vi "Main HMI.vi"() -> ()   [LabVIEW 2014]
uses:
  Controls/Icon Arrow H.ctl
  Controls/Icon Line H.ctl
  Controls/Icon Switch H.ctl
  Controls/Meter SOC.ctl
  Controls/Icon Load.ctl
  Controls/Icon Battery.ctl
  Controls/Icon Inverter.ctl
  Controls/Icon Generator.ctl
  Controls/Icon PV.ctl
  Controls/HMI Tab.ctl
  Controls/Alarm Display.ctl
  Controls/Icon Line V.ctl
  Controls/Icon Arrow V.ctl
  Controls/Icon Switch V.ctl
  Controls/Interface Data.ctl
  Controls/Gen Data.ctl
  Controls/HMI State.ctl
  Controls/Alarms Data.ctl
  Controls/LogState.ctl
panel:
  out "Alarms Page":bool=TRUE
  out "Main Page":bool=TRUE
  out "Tab Control":T1
  out "Arrow 2":T2
  out "Arrow 1":T2
  out "Line Inverter3":T3
  out "Line Inverter2":T4
  out "Arrow 19":T5
  out "Arrow 18":T5
  out "Arrow 17":T5
  out "Arrow 16":T5
  out "Arrow 15":T5
  out "Arrow 12":T5
  out "Arrow 11":T5
  out "Line Gen Both":T4
  out "Line Inverter1":T3
  out "Line Gen W 3":T4
  out "Line Gen E 4":T4
  out "SOH":dbl format="%2.0f %"
  out "Gen East Hours":dbl format="%2.0f Hrs"
  out "Switch Gen E":T6
  out "Gen West Hours":dbl format="%2.0f Hrs"
  out "Gen East":T7
  out "Line Gen E 2":T4
  out "Load":T8
  out "Line Load":T4
  out "Arrow 10":T5
  out "Arrow 9":T5
  out "Switch Gen W":T6
  out "Switch Battery":T6
  out "Line Gen W 2":T4
  out "Gen West":T7
  out "SOC":T9 scale=0.0..100.0 scale format="%3.0f %"
  out "Batteries":T10
  out "Inverter":T11
  out "Line Batteries 1":T4
  out "Line Batteries 2":T4
  out "Switch PV":T6
  out "PV":T12
  out "Line PV":T4
  out "Line PV2":T4
  out "Solar kW":dbl format="%2.1f kW"
  out "Line Gen E 3":T3
  out "Line PV3":T3
  out "Switch Inverter":T13
  out "Converter Version":string
  out "RT Version":string
  out "FPGA Version":string
  out "HMI Version":string
  in  "Exit Program":bool
  out "InterfaceData":T14 {"GenEast"."TotalFuel(L)" format="%.2f"; "GenEast"."FuelRate(L/H)" format="%.2f"; "GenEast"."ApparentPower(VA)" format="%.2f"; "GenEast"."BattVoltage(V)" format="%.2f"; "GenEast"."Freq(Hz)" format="%.2f"; "GenEast"."RunHours(hr)" format="%.2f"; "GenEast"."PowerFactor" format="%.2f"; "GenEast"."ReactivePower(VAR)" format="%.2f"; "GenEast"."ActivePower(W)" format="%.2f"; "GenWest"."TotalFuel(L)" format="%.2f"; "GenWest"."FuelRate(L/H)" format="%.2f"; "GenWest"."ApparentPower(VA)" format="%.2f"; "GenWest"."BattVoltage(V)" format="%.2f"; "GenWest"."Freq(Hz)" format="%.2f"; "GenWest"."RunHours(hr)" format="%.2f"; "GenWest"."PowerFactor" format="%.2f"; "GenWest"."ReactivePower(VAR)" format="%.2f"; "GenWest"."ActivePower(W)" format="%.2f"; "Converter Alarms 2" format="%016b"; "Converter Faults 2" format="%016b"; "Controller Faults" format="%016b"; "System Status" format="%016b"; "Converter Alarms 1" format="%016b"; "Converter Faults 1" format="%016b"; "Solar Faults" format="%016b"; "ES Rack 10 Alarms" format="%016b"; "ES Rack 9 Alarms" format="%016b"; "ES Rack 8 Alarms" format="%016b"; "ES Rack 7 Alarms" format="%016b"; "ES Rack 6 Alarms" format="%016b"; "ES Rack 5 Alarms" format="%016b"; "ES Rack 4 Alarms" format="%016b"; "ES Rack 3 Alarms" format="%016b"; "ES Rack 2 Alarms" format="%016b"; "ES Rack 1 Alarms" format="%016b"; "ES System Alarms" format="%016b"; "System Faults" format="%016b"; "ES Rack 10 Faults" format="%016b"; "ES Rack 9 Faults" format="%016b"; "ES Rack 8 Faults" format="%016b"; "ES Rack 7  Faults" format="%016b"; "ES Rack 6 Faults" format="%016b"; "ES Rack 5 Faults" format="%016b"; "ES Rack 4 Faults" format="%016b"; "ES Rack 3 Faults" format="%016b"; "ES Rack 2 Faults" format="%016b"; "ES Rack 1 Faults" format="%016b"; "ES System Faults" format="%016b"}
  out "Alarms List":T16
  in  "Clear Alarms":bool
  out "Event Log Error":bool
  out "Data Log Error":bool
  out "GENERATOR EAST":T17(ring)
  out "GENERATOR WEST":T17(ring)
  out "POWER SYSTEM STATUS":T18(ring)
  out "SOLAR ARRAY":T19(ring)
  out "BATTERY ARRAY":T17(ring)
  out "Status Page":bool=TRUE
  out "Connection Error":bool
  out "System Status":string
  out "Diagnostics Page":bool=TRUE
  out "Fault Banner":bool
  out "Alarm Banner":bool
  # "Manual\nBreaker"
  # "Manual\nBreaker"
  # "Manual\nBreaker"
  # "Facility"
  # "Manual\nBreaker"
  # "Service Entrance Switchboard"
  # "Generator Housing"
  # "Solar Array Box"
  # "Manual\nBreaker"
  # "Battery Connex/Solid State Generator"
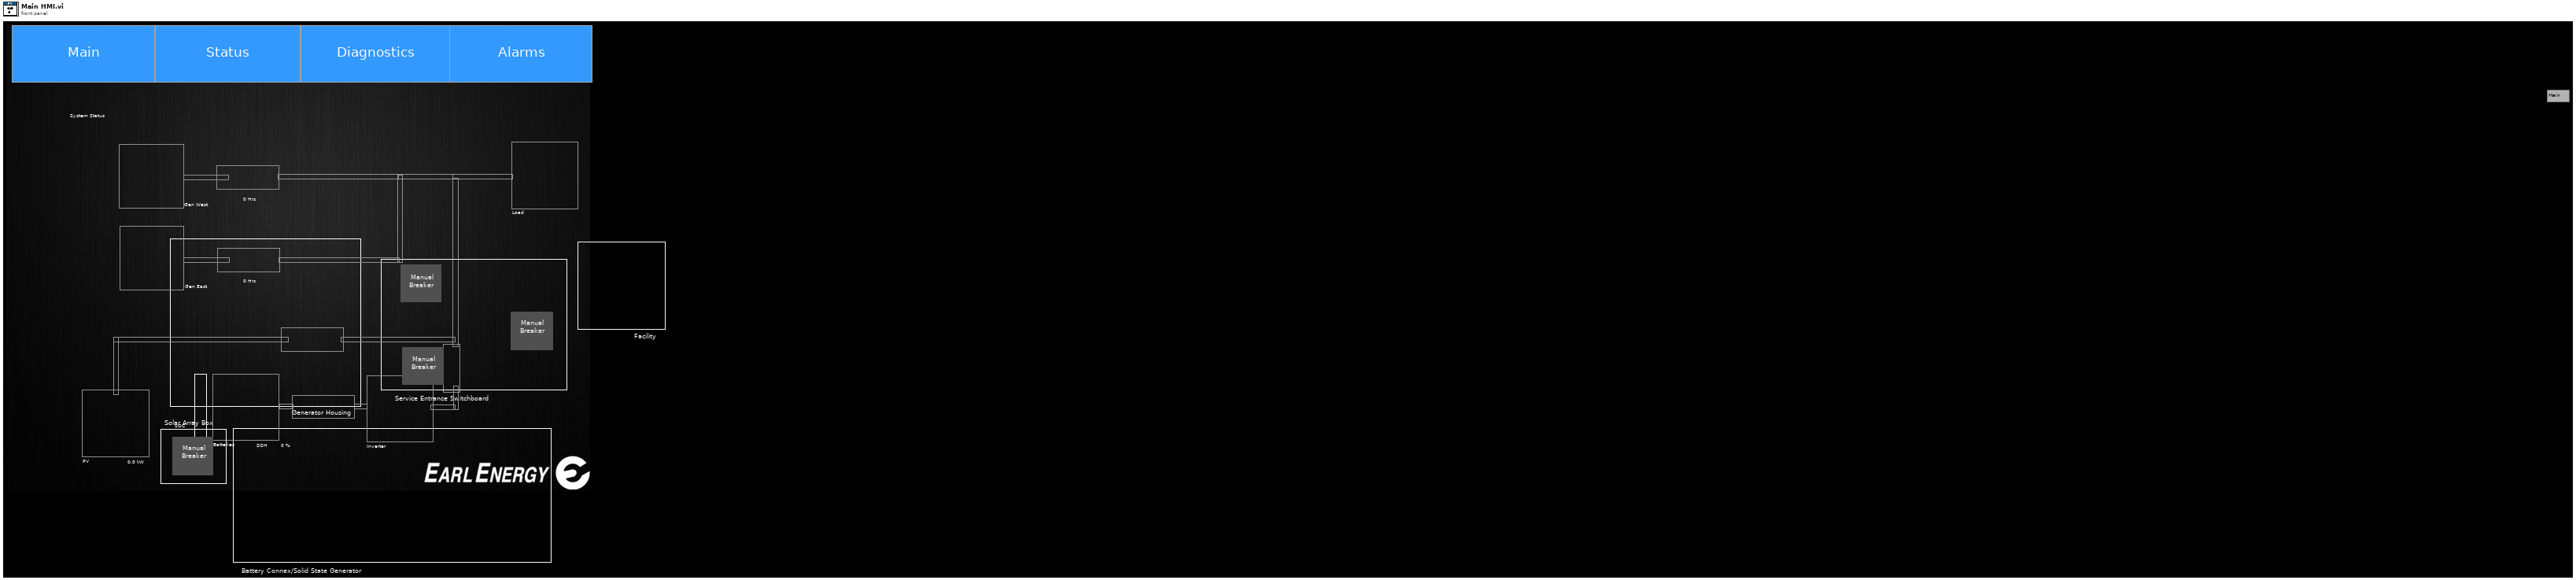
[diagram p1: front panel]
types:
  T1 = typedef "HMI Tab.ctl" = enum32{"Main", "Diagnostics", "Alarms", "Status"}
  T2 = typedef "Icon Arrow V.ctl" = bool
  T3 = typedef "Icon Line V.ctl" = bool
  T4 = typedef "Icon Line H.ctl" = bool
  T5 = typedef "Icon Arrow H.ctl" = bool
  T6 = typedef "Icon Switch H.ctl" = bool
  T7 = typedef "Icon Generator.ctl" = bool
  T8 = typedef "Icon Load.ctl" = bool
  T9 = typedef "Meter SOC.ctl" = dbl
  T10 = typedef "Icon Battery.ctl" = bool
  T11 = typedef "Icon Inverter.ctl" = bool
  T12 = typedef "Icon PV.ctl" = bool
  T13 = typedef "Icon Switch V.ctl" = bool
  T14 = typedef "Interface Data.ctl" = cluster{"SSG AC Current":i16, "SSG AC Voltage":i16, "SSC Active Power":i16, "SSG Reactive Power":i16, "SSG Apparent Power":i16, "SSG Frequency":i16, "ES SOC":i16, "ES SOH":i16, "ES Voltage":i16, "ES # Strings":i16, "ES # Cycles":i16, "ES Temperature":i16, "PC Temperature":i16, "Solar Active Power":i16, "Converter Version":i16, "Controller Version":i16, "System Status":i16, "System Faults":i16, "Controller Faults":i16, "ES System Faults":i16, "ES System Alarms":i16, "Converter Faults 1":i16, "Converter Faults 2":i16, "Converter Alarms 1":i16, "Converter Alarms 2":i16, "Solar Faults":i16, "ES Rack 1 Faults":i16, "ES Rack 2 Faults":i16, "ES Rack 3 Faults":i16, "ES Rack 4 Faults":i16, "ES Rack 5 Faults":i16, "ES Rack 6 Faults":i16, "ES Rack 7  Faults":i16, "ES Rack 8 Faults":i16, "ES Rack 9 Faults":i16, "ES Rack 10 Faults":i16, "ES Rack 1 Alarms":i16, "ES Rack 2 Alarms":i16, "ES Rack 3 Alarms":i16, "ES Rack 4 Alarms":i16, "ES Rack 5 Alarms":i16, "ES Rack 6 Alarms":i16, "ES Rack 7 Alarms":i16, "ES Rack 8 Alarms":i16, "ES Rack 9 Alarms":i16, "ES Rack 10 Alarms":i16, "GenWest":T15, "GenEast":T15}
  T15 = typedef "Gen Data.ctl" = cluster{"Warning":bool, "System Fault":bool, "Com Fault":bool, "Alarms":string[], "ControllerMode":u16, "ActivePower(W)":i32, "ReactivePower(VAR)":i32, "PowerFactor":dbl, "RunHours(hr)":dbl, "Freq(Hz)":dbl, "BattVoltage(V)":dbl, "ApparentPower(VA)":i32, "FuelRate(L/H)":dbl, "TotalFuel(L)":u32, "IsRunning":bool}
  T16 = typedef "Alarm Display.ctl" = string[]
  T17 = enum16{"OFF", "ON", "Charging", "Discharging", "Call Maint", "Faulted"}
  T18 = enum16{"OFF", "ON", "Charging", "Discharging", "Call Maint", "Faulted", "NORMAL"}
  T19 = enum16{"ON", "OFF", "Charging", "Discharging", "Call Maint", "Faulted"}
  T20 = typedef "LogState.ctl" = enum16{"Remove Null Data", "Rotate Log", "Log Data", "Wait", "Close File", "Open File"}
  T21 = typedef "Alarms Data.ctl" = cluster{"Message Array":string[], "Fault Array":bool[], "Alarm Array":bool[]}
  T22 = typedef "HMI State.ctl" = enum16{"Timeout", "Go to Main Page", "Go to Status Page", "Go to Diagnostics Page", "Go to Alarms Page", "Shutdown", "Startup", "Spot Gen - Charging", "Spot Gen - Discharging", "Fault", "Alarm"}
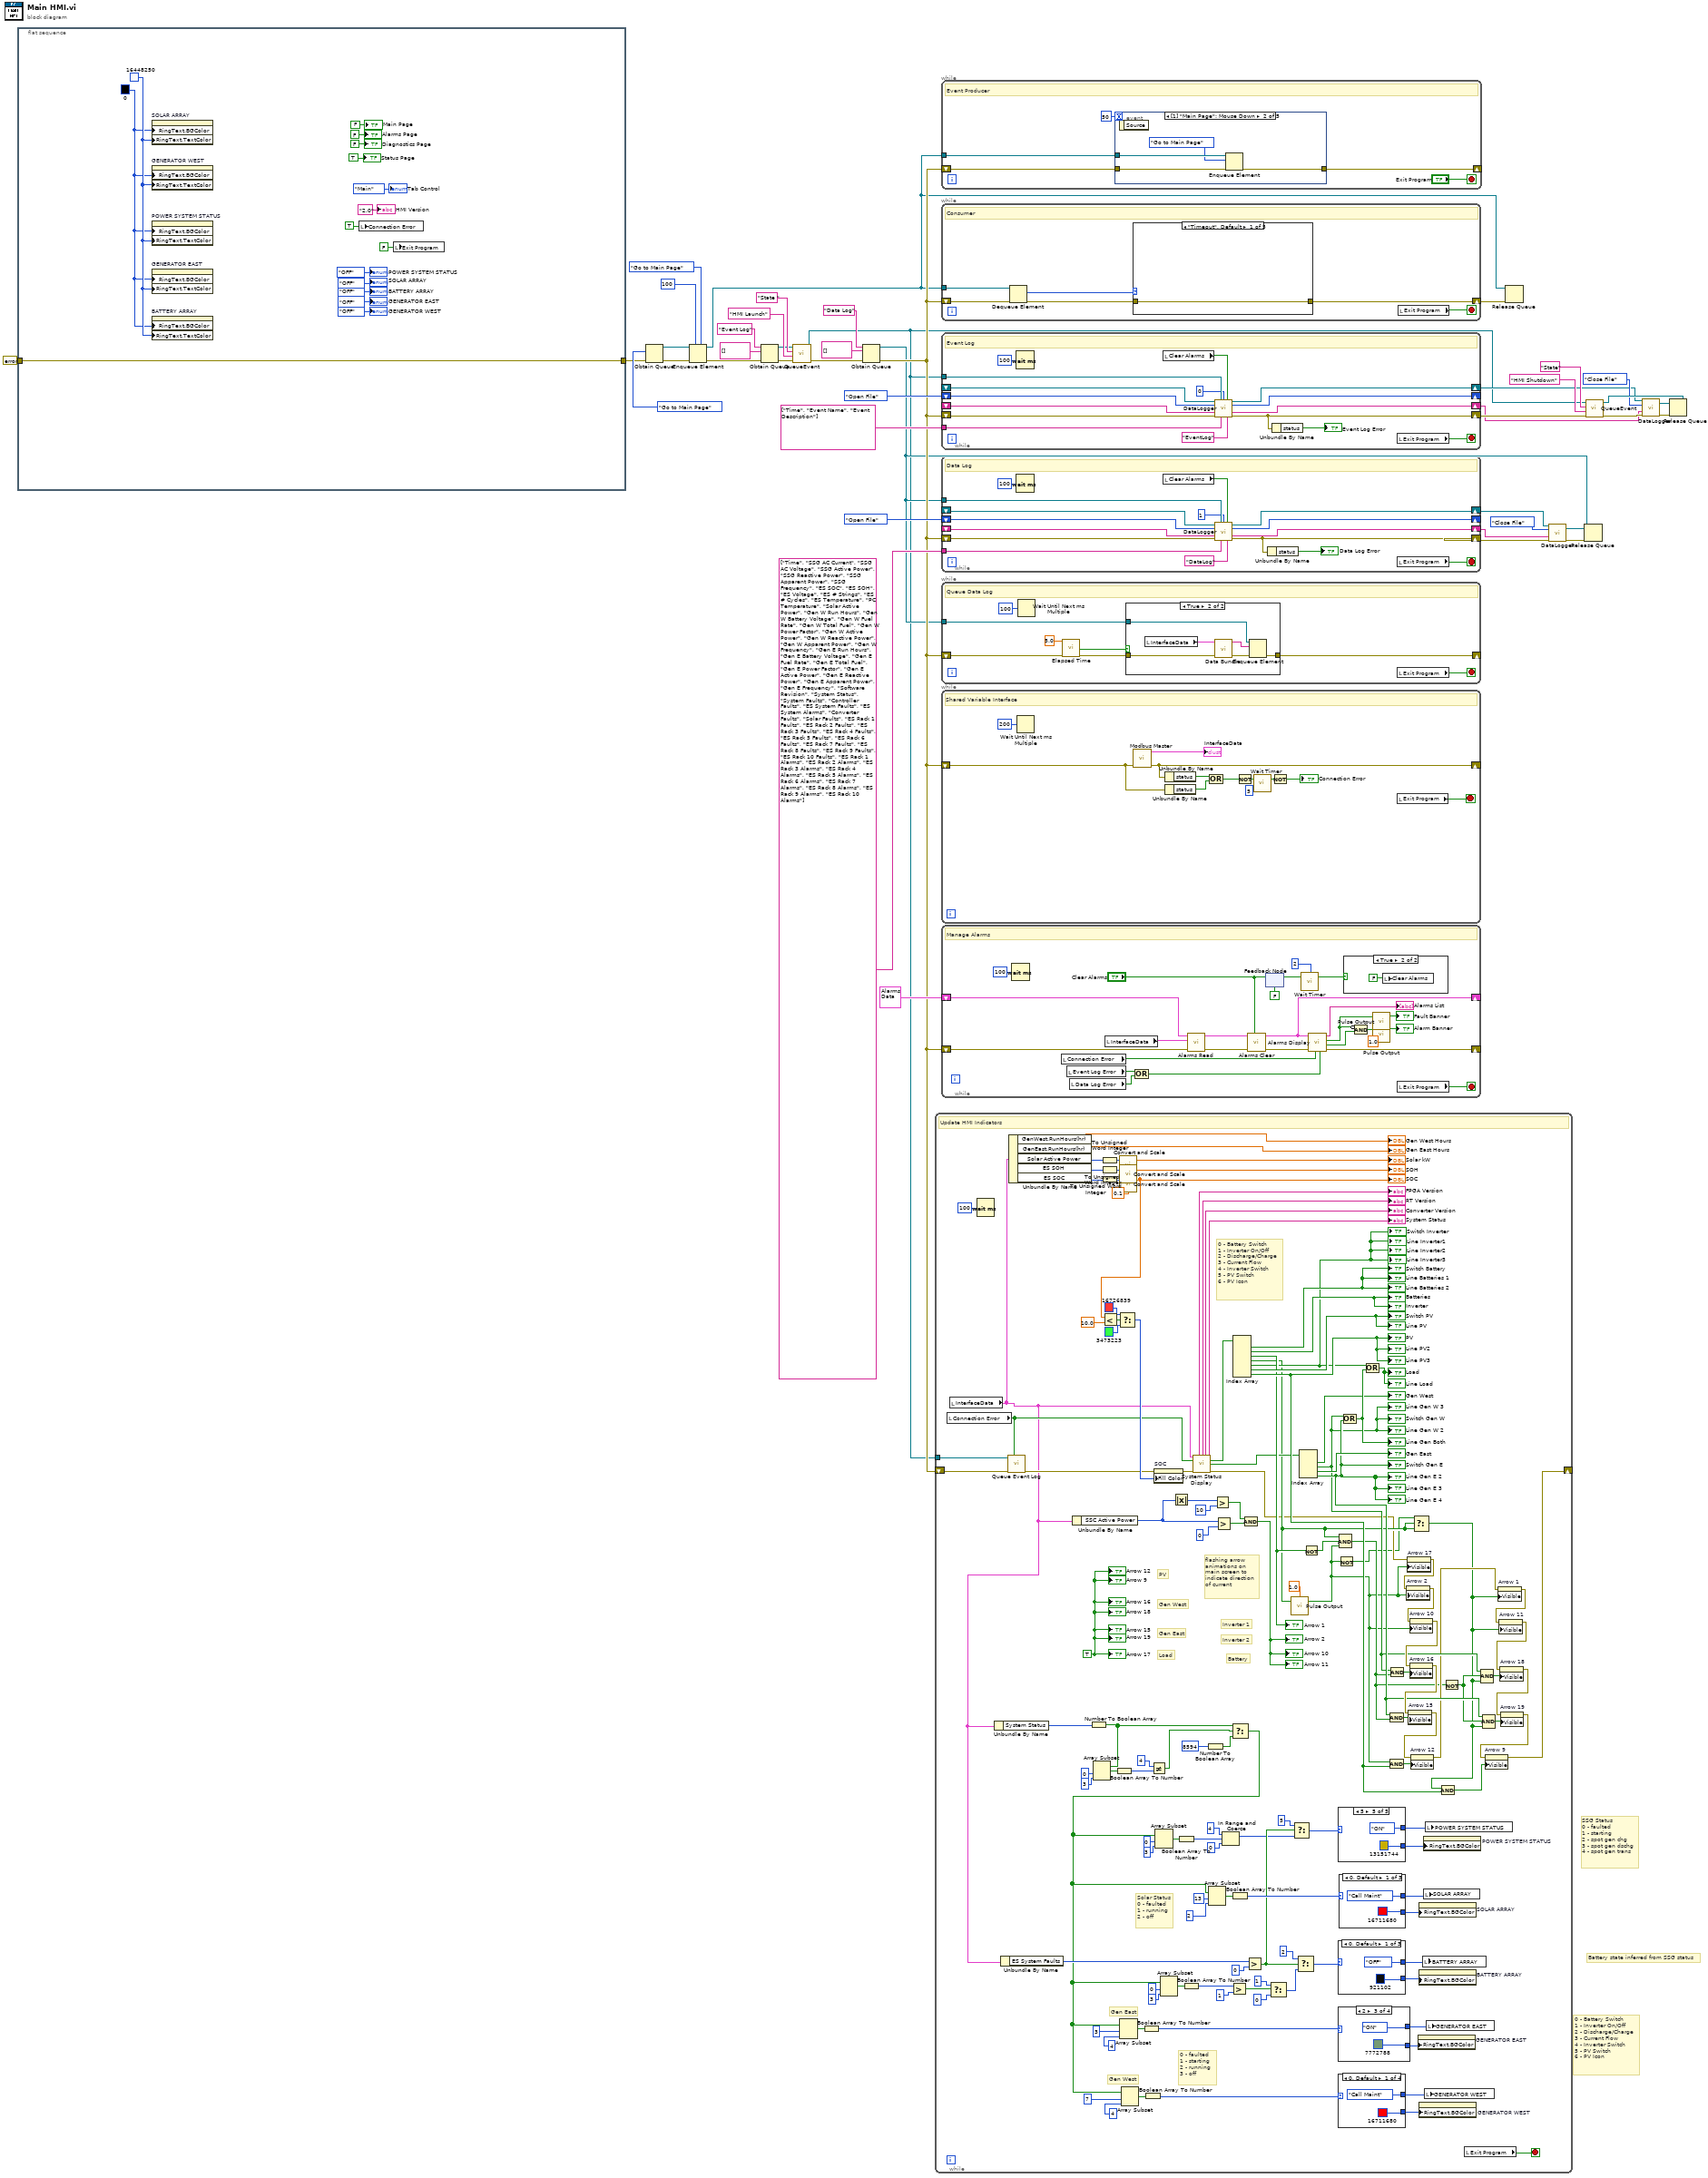
[diagram p0: block diagram]
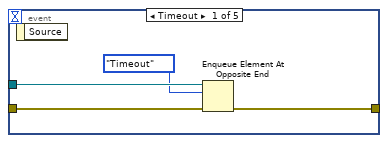
[diagram p4: hidden frame]
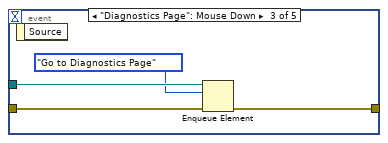
[diagram p5: hidden frame]
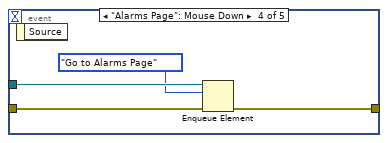
[diagram p6: hidden frame]
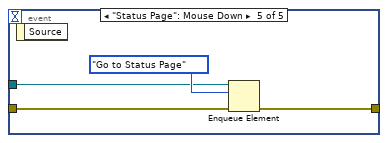
[diagram p7: hidden frame]
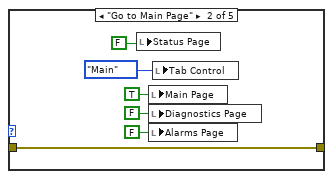
[diagram p8: hidden frame]
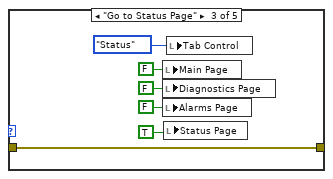
[diagram p9: hidden frame]
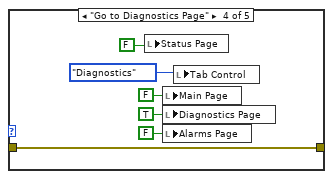
[diagram p10: hidden frame]
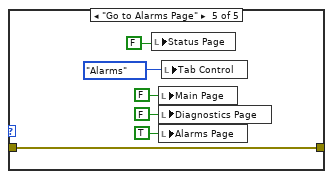
[diagram p11: hidden frame]
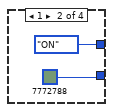
[diagram p12: hidden frame]
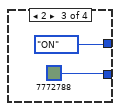
[diagram p13: hidden frame]
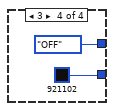
[diagram p14: hidden frame]
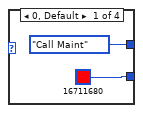
[diagram p15: hidden frame]
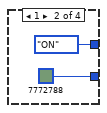
[diagram p16: hidden frame]
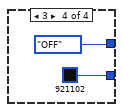
[diagram p17: hidden frame]
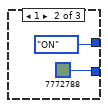
[diagram p18: hidden frame]
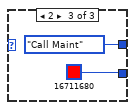
[diagram p19: hidden frame]
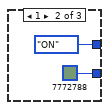
[diagram p20: hidden frame]
diagram:
  # "Battery state inferred from SSG status"
  # "SSG Status\n0 - faulted\n1 - starting\n2 - spot gen chg\n3 - spot gen dschg\n4 - spot gen trans"
  # "0 - Battery Switch\n1 - Inverter On/Off\n2 - Discharge/Charge\n3 - Current Flow\n4 - Inverter Switch\n5 - PV Switch\n6 - PV Icon"
  n1 = flat-sequence {
    tunnel: errorcluster {"status"=FALSE, "code"=0, "source"=""} ("error out") -> [w46]
    tunnel: [w46] -> w2
    frame #0 {
      w42 = u32 0 ("Fill Color")
      w43 = u32 16448250 ("Fill Color")
      n2 = property on="SOLAR ARRAY" class="Enum (strict)"("RingText.BGColor"=w42, "RingText.TextColor"=w43) -> ()  [unwired: 2 in, 2 out]
      n3 = property on="GENERATOR WEST" class="Enum (strict)"("RingText.BGColor"=w42, "RingText.TextColor"=w43) -> ()  [unwired: 2 in, 2 out]
      n4 = property on="POWER SYSTEM STATUS" class="Enum (strict)"("RingText.BGColor"=w42, "RingText.TextColor"=w43) -> ()  [unwired: 2 in, 2 out]
      n5 = property on="GENERATOR EAST" class="Enum (strict)"("RingText.BGColor"=w42, "RingText.TextColor"=w43) -> ()  [unwired: 2 in, 2 out]
      n6 = property on="BATTERY ARRAY" class="Enum (strict)"("RingText.BGColor"=w42, "RingText.TextColor"=w43) -> ()  [unwired: 2 in, 2 out]
      n7 = local write "Connection Error"(TRUE ("Connection Error")) -> ()
      n8 = local write "Exit Program"(FALSE ("Exit Program")) -> ()
      "Tab Control" <- HMI_Tab."Main" ("Tab Control")
      "Main Page" <- FALSE ("Main Page")
      "Alarms Page" <- FALSE ("Alarms Page")
      "Diagnostics Page" <- FALSE ("Diagnostics Page")
      "HMI Version" <- "2.0" ("HMI Version")
      "Status Page" <- TRUE ("Status Page")
      "POWER SYSTEM STATUS" <- T18."OFF" ("Power System Status")
      "SOLAR ARRAY" <- T19."OFF" ("Solar Array")
      "BATTERY ARRAY" <- T17."OFF" ("Battery Array")
      "GENERATOR EAST" <- T17."OFF" ("Generater East")
      "GENERATOR WEST" <- T17."OFF" ("Generator West")
    }
  }
  n9 = Obtain Queue(element data type=HMI_State."Go to Main Page" ("State"), error in (no error)=w2) -> (queue out=w40:refnum<queue>, error out=w39:errorcluster)  [unwired: 3 in, 1 out]
  n10 = Enqueue Element(queue=w40, element=HMI_State."Go to Main Page", timeout in ms (-1)=100, error in (no error)=w39) -> (queue out=w1:refnum<queue>, error out=w21:errorcluster)  [unwired: 1 out]
  n11 = Obtain Queue(name (unnamed)="Event Log", element data type=string[] [], error in (no error)=w21) -> (queue out=w23:refnum<queue>, error out=w22:errorcluster)  [unwired: 2 in, 1 out]
  n12 = call "QueueEvent.vi"("Error In"=w22, "Event Description"="HMI Launch", "Event Name"="State ", "Queue In"=w23) -> ("Error Out"=w26:errorcluster, "Queue Out"=w3:refnum<queue>)  [unwired: 6 in]
  n13 = Obtain Queue(name (unnamed)="Data Log", element data type=string[] [], error in (no error)=w26) -> (queue out=w4:refnum<queue>, error out=w5:errorcluster)  [unwired: 2 in, 1 out]
  n14 = while {
    shift-right: [w138] -> _
    shift-left: w5 -> [w177]
    tunnel: w3 -> [w176]
    stop <- w189 stop-if-true
    w164 = T5 TRUE ("Arrow 17")
    w170 = 0.1 ("Scale Value")
    # "Solar Status\n0 - faulted\n1 - running\n2 - off"
    # "0 - faulted\n1 - starting\n2 - running \n3 - off"
    # "Gen West"
    # "Gen East"
    # "0 - Battery Switch\n1 - Inverter On/Off\n2 - Discharge/Charge\n3 - Current Flow\n4 - Inverter Switch\n5 - PV Switch\n6 - PV Icon"
    # "Inverter 2"
    # "Inverter 1"
    # "Battery"
    # "PV"
    # "Load"
    # "Gen East"
    # "Gen West"
    # "flashing arrow \nanimations on \nmain screen to\nindicate direction\nof current"
    # "Update HMI Indicators"
    n15 = local read "Connection Error"() -> (w128:bool)
    n16 = local read "InterfaceData"() -> (w58:T14)
    n17 = Wait (ms)(milliseconds to wait=u32 100) -> ()  [unwired: 1 out]
    n18 = Unbundle By Name(w58) -> ("System Status"=w71:i16)
    n19 = Unbundle By Name(w58) -> ("ES System Faults"=w110:i16)
    n20 = call "Queue Event Log.vi"("Connection Error"=w128, "Error In"=w177, "Event Log Queue"=w176) -> ("Error Out"=w104:errorcluster)  [unwired: 8 in]
    n21 = Unbundle By Name(w58) -> ("GenWest.RunHours(hr)"=→"Gen West Hours":dbl, "GenEast.RunHours(hr)"=→"Gen East Hours":dbl, "Solar Active Power"=w169:i16, "ES SOH"=w175:i16, "ES SOC"=w174:i16)
    n22 = Unbundle By Name(w58) -> ("SSC Active Power"=w130:i16)
    n23 = Number To Boolean Array(number=w71) -> (Boolean array=w75:bool[])
    n24 = Array Subset(array=w75, index=0, length=3) -> (w77:bool[])
    n25 = To Unsigned Word Integer(number=w174) -> (unsigned 16bit integer=w173:u16)
    n26 = To Unsigned Word Integer(number=w169) -> (unsigned 16bit integer=w171:u16)
    n27 = To Unsigned Word Integer(number=w175) -> (unsigned 16bit integer=w172:u16)
    n28 = Boolean Array To Number(Boolean array=w77) -> (number=w76:u32)
    n29 = call "Convert and Scale.vi"("Number In"=w171, "Scale Value"=w170) -> ("Converter Number Out"=→"Solar kW":dbl)  [unwired: 3 in]
    n30 = call "Convert and Scale.vi"("Number In"=w172, "Scale Value"=w170) -> ("Converter Number Out"=→"SOH":dbl)  [unwired: 3 in]
    n31 = call "Convert and Scale.vi"("Number In"=w173, "Scale Value"=w170) -> ("Converter Number Out"=w70:dbl)  [unwired: 3 in]
    "SOC" <- w70
    n32 = Less?(x=w70, y=10.0) -> (x < y?=w179:bool)
    n33 = Select(t=u32 16726839 ("Fill Color"), s=w179, f=u32 3473223 ("Fill Color")) -> (s? t:f=w182:u32)
    n34 = Not Equal?(x=u32 4, y=w76) -> (x != y?=w74:bool)
    n35 = property on="SOC" class="Slide (strict)"(error in=w104, "Fill Color"=w182) -> (error out=w183:errorcluster)  [unwired: 1 in, 1 out]
    n36 = Absolute Value(x=w130) -> (abs(x)=w133:i16)
    n37 = call "System Status Display.vi"("InterfaceData"=w58, "Connection Error"=w128, "Error In"=w183) -> ("FPGA Version"=→"FPGA Version":string, "RT Version"=→"RT Version":string, "Converter Version"=→"Converter Version":string, "System Status"=→"System Status":string, "System Status Data"=w184:bool[], "Gen Status Data"=w134:bool[], "Error Out"=w122:errorcluster)  [unwired: 6 in]
    n38 = Number To Boolean Array(number=i16 8594) -> (Boolean array=w73:bool[])
    n39 = Greater?(x=w133, y=i16 10) -> (0:w158:bool)
    n40 = Greater?(x=w130, y=i16 0) -> (0:w157:bool)
    n41 = Select(t=w75, s=w74, f=w73) -> (s? t:f=w80:bool[])
    n42 = Array Subset(array=w80, index=3, length=4) -> (w94:bool[])
    n43 = Array Subset(array=w80, index=7, length=4) -> (w92:bool[])
    n44 = Boolean Array To Number(Boolean array=w94) -> (number=w93:u8)
    n45 = Boolean Array To Number(Boolean array=w92) -> (number=w91:u8)
    n46 = Array Subset(array=w80, index=0, length=3) -> (w99:bool[])
    n47 = Array Subset(array=w80, index=0, length=3) -> (w87:bool[])
    n48 = Boolean Array To Number(Boolean array=w99) -> (number=w64:u32)
    n49 = Boolean Array To Number(Boolean array=w87) -> (number=w85:u32)
    n50 = Array Subset(array=w80, index=13, length=2 ("index")) -> (w103:bool[])
    n51 = In Range and Coerce(upper limit=u32 4, x=w64, lower limit=u32 0) -> (coerced(x)=w63:u32)  [unwired: 1 out]
    n52 = Greater?(x=w85, y=i16 1) -> (0:w86:bool)
    n53 = Boolean Array To Number(Boolean array=w103) -> (number=w102:u32)
    n54 = Index Array(array=w184) -> (element #1=→"Switch Battery" →"Line Batteries 2" →"Line Batteries 1":bool, element #2=→"Inverter" →"Batteries":bool, element #3=w153:bool, element #4=w125:bool, element #5=w137:bool, element #6=→"Line PV" →"Switch PV":bool, element #7=w160:bool)  [unwired: 7 in]
    "Line PV2" <- w160
    "PV" <- w160
    "Line Inverter1" <- w137
    "Line PV3" <- w160
    "Line Inverter2" <- w137
    "Line Inverter3" <- w137
    "Arrow 1" <- w153
    "Switch Inverter" <- w137
    n55 = Compound Arithmetic op=AND(w158, w157) -> (→"Arrow 10" →"Arrow 11" →"Arrow 2":bool)
    n56 = Greater?(x=w110, y=i16 0) -> (0:w67:bool)
    n57 = Select(t=u32 1, s=w86, f=u32 0) -> (s? t:f=w83:u32)
    n58 = call "Pulse Output.vi"("Boolean In"=w125, "Time Target (s)"=1.0) -> ("Boolean Out"=w123:bool)  [unwired: 3 in]
    n59 = Select(t=u32 5, s=w67, f=w63) -> (s? t:f=w66:u32)
    n60 = Select(t=i16 2, s=w67, f=w83) -> (s? t:f=w107:u32)
    n61 = Index Array(array=w134) -> (element #1=→"Gen West":bool, element #2=w135:bool, element #3=→"Gen East":bool, element #4=w136:bool)  [unwired: 4 in]
    "Line Gen E 2" <- w136
    "Line Gen E 3" <- w136
    "Switch Gen E" <- w136
    "Switch Gen W" <- w135
    "Line Gen W 2" <- w135
    "Line Gen W 3" <- w135
    "Line Gen E 4" <- w136
    n62 = Not(x=w153) -> (.not. x?=w154:bool)
    n63 = Not(x=w123) -> (.not. x?=w121:bool)
    n64 = case shown="5" w66 {
      tunnel: [T18."Call Maint" ("POWER SYSTEM STATUS") T18."ON" ("POWER SYSTEM STATUS") T18."NORMAL" ("POWER SYSTEM STATUS") T18."NORMAL" ("POWER SYSTEM STATUS") T18."ON" ("POWER SYSTEM STATUS")] -> w115
      tunnel: [u32 16711680 u32 7772788 u32 7772788 u32 7772788 u32 13151744] -> w120
      frame 0, Default {
      }
      frame 1 {
      }
      frame 2, 3 {
      }
      frame 4 {
      }
      frame 5 {
      }
    }
    n65 = case shown="0, Default" w107 {
      tunnel: [u32 921102 u32 7772788 u32 16711680] -> w118
      tunnel: [T17."OFF" ("Battery Array") T17."ON" ("BATTERY ARRAY") T17."Call Maint" ("BATTERY ARRAY")] -> w113
      frame 0, Default {
      }
      frame 1 {
      }
      frame 2 {
      }
    }
    n66 = case shown="2" w93 {
      tunnel: [u32 16711680 u32 7772788 u32 7772788 u32 921102] -> w117
      tunnel: [T17."Call Maint" ("Generater East") T17."ON" ("Generater East") T17."ON" ("Generater East") T17."OFF" ("Generater East")] -> w111
      frame 0, Default {
      }
      frame 1 {
      }
      frame 2 {
      }
      frame 3 {
      }
    }
    n67 = case shown="0, Default" w91 {
      tunnel: [u32 16711680 u32 7772788 u32 7772788 u32 921102] -> w116
      tunnel: [T17."Call Maint" ("Generator West") T17."ON" ("Generator West") T17."ON" ("Generator West") T17."OFF" ("Generator West")] -> w112
      frame 0, Default {
      }
      frame 1 {
      }
      frame 2 {
      }
      frame 3 {
      }
    }
    n68 = Compound Arithmetic op=AND(w125, w154, w123) -> (w127:bool)
    n69 = case shown="0, Default" w102 {
      tunnel: [u32 16711680 u32 7772788 u32 921102] -> w119
      tunnel: [T19."Call Maint" ("SOLAR ARRAY") T19."ON" ("SOLAR ARRAY") T19."OFF" ("SOLAR ARRAY")] -> w114
      frame 0, Default {
      }
      frame 1 {
      }
      frame 2 {
      }
    }
    n70 = Compound Arithmetic op=OR(w135, w136) -> (w165:bool)
    "Line Gen Both" <- w165
    n71 = Compound Arithmetic op=OR(w137, w165) -> (→"Load" →"Line Load":bool)
    n72 = Compound Arithmetic op=AND(w136, w127) -> (w150:bool)
    n73 = Compound Arithmetic op=AND(w123, w160) -> (w162:bool)
    n74 = Compound Arithmetic op=AND(w135, w127) -> (w140:bool)
    n75 = property on="Arrow 17" class="Bool (strict)"(error in=w122, "Visible"=w123) -> (error out=w132:errorcluster)  [unwired: 1 in, 1 out]
    n76 = property on="Arrow 2" class="Bool (strict)"(error in=w132, "Visible"=w123) -> (error out=w166:errorcluster)  [unwired: 1 in, 1 out]
    n77 = property on="Arrow 10" class="Bool (strict)"(error in=w166, "Visible"=w123) -> (error out=w146:errorcluster)  [unwired: 1 in, 1 out]
    n78 = property on="Arrow 16" class="Bool (strict)"(error in=w146, "Visible"=w140) -> (error out=w145:errorcluster)  [unwired: 1 in, 1 out]
    n79 = property on="Arrow 15" class="Bool (strict)"(error in=w145, "Visible"=w150) -> (error out=w144:errorcluster)  [unwired: 1 in, 1 out]
    n80 = property on="Arrow 12" class="Bool (strict)"(error in=w144, "Visible"=w162) -> (error out=w131:errorcluster)  [unwired: 1 in, 1 out]
    n81 = Select(t=w121, s=w125, f=w125) -> (s? t:f=w124:bool)
    n82 = property on="GENERATOR EAST" class="Enum (strict)"("RingText.BGColor"=w117) -> ()  [unwired: 2 in, 2 out]
    n83 = property on="SOLAR ARRAY" class="Enum (strict)"("RingText.BGColor"=w119) -> ()  [unwired: 2 in, 2 out]
    n84 = property on="BATTERY ARRAY" class="Enum (strict)"("RingText.BGColor"=w118) -> ()  [unwired: 2 in, 2 out]
    n85 = property on="GENERATOR WEST" class="Enum (strict)"("RingText.BGColor"=w116) -> ()  [unwired: 2 in, 2 out]
    n86 = local write "BATTERY ARRAY"(w113) -> ()
    n87 = property on="POWER SYSTEM STATUS" class="Enum (strict)"("RingText.BGColor"=w120) -> ()  [unwired: 2 in, 2 out]
    n88 = local write "SOLAR ARRAY"(w114) -> ()
    n89 = local write "GENERATOR WEST"(w112) -> ()
    n90 = local write "POWER SYSTEM STATUS"(w115) -> ()
    n91 = local write "GENERATOR EAST"(w111) -> ()
    n92 = Compound Arithmetic op=AND(w124, w160) -> (w159:bool)
    n93 = Not(x=w127) -> (.not. x?=w126:bool)
    n94 = local read "Exit Program"() -> (w189:bool)
    n95 = Compound Arithmetic op=AND(w135, w126, w124) -> (w152:bool)
    n96 = Compound Arithmetic op=AND(w136, w126, w124) -> (w151:bool)
    n97 = property on="Arrow 1" class="Bool (strict)"(error in=w131, "Visible"=w124) -> (error out=w143:errorcluster)  [unwired: 1 in, 1 out]
    n98 = property on="Arrow 11" class="Bool (strict)"(error in=w143, "Visible"=w124) -> (error out=w142:errorcluster)  [unwired: 1 in, 1 out]
    n99 = property on="Arrow 18" class="Bool (strict)"(error in=w142, "Visible"=w152) -> (error out=w141:errorcluster)  [unwired: 1 in, 1 out]
    n100 = property on="Arrow 19" class="Bool (strict)"(error in=w141, "Visible"=w151) -> (error out=w139:errorcluster)  [unwired: 1 in, 1 out]
    n101 = property on="Arrow 9" class="Bool (strict)"(error in=w139, "Visible"=w159) -> (error out=w138:errorcluster)  [unwired: 1 in, 1 out]
    "Arrow 9" <- w164
    "Arrow 12" <- w164
    "Arrow 17" <- w164
    "Arrow 16" <- w164
    "Arrow 15" <- w164
    "Arrow 18" <- w164
    "Arrow 19" <- w164
  }
  n102 = while {
    shift-right: [w229] -> _
    shift-left: w5 -> [w238]
    stop <- w240 stop-if-true
    # "Shared Variable Interface"
    n103 = Wait Until Next ms Multiple(millisecond multiple=u32 200 ("milliseconds to wait")) -> ()  [unwired: 1 out]
    n104 = call "Modbus Master.vi"("Error In"=w238) -> ("Error Out"=w229:errorcluster, "InterfaceData"=→"InterfaceData":T14)  [unwired: 9 in]
    n105 = Unbundle By Name(w229) -> ("status"=w237:bool)
    n106 = Unbundle By Name(w238) -> ("status"=w236:bool)
    n107 = Compound Arithmetic op=OR(w237, w236) -> (w232:bool)
    n108 = Not(x=w232) -> (.not. x?=w234:bool)
    n109 = call "Wait Timer.vi"("Boolean In"=w234, "Timer"=u32 5) -> ("Boolean Out"=w235:bool)  [unwired: 3 in]
    n110 = Not(x=w235) -> (.not. x?=→"Connection Error":bool)
    n111 = local read "Exit Program"() -> (w240:bool)
  }
  n112 = while {
    tunnel: w1 -> [w244]
    shift-right: [w243] -> _
    shift-left: w5 -> [w245]
    stop <- "Exit Program" stop-if-true
    # "Event Producer"
    n113 = event shown="[1] \"Main Page\": Mouse Down" {
      selector: _ -> [_ _ _ _ _]
      dyn-events: _ -> [_ _ _ _ _]
      timeout: 50 -> [_ _ _ _ _]
      tunnel: w245 -> [w249 w253 w257 w261 w264]
      tunnel: w244 -> [w247 w252 w256 w260 w262]
      tunnel: [w248 w250 w254 w258 w263] -> w243
      event Timeout {
        n114 = event-data() -> ()  [unwired: 1 in, 1 out]
        n115 = Enqueue Element At Opposite End(queue=w247, element=HMI_State."Timeout", error in (no error)=w249) -> (error out=w248:errorcluster)  [unwired: 1 in, 2 out]
      }
      event "Main Page": Mouse Down {
        n116 = event-data() -> ()  [unwired: 1 in, 1 out]
        n117 = Enqueue Element(queue=w252, element=HMI_State."Go to Main Page", error in (no error)=w253) -> (error out=w250:errorcluster)  [unwired: 1 in, 2 out]
      }
      event "Diagnostics Page": Mouse Down {
        n118 = event-data() -> ()  [unwired: 1 in, 1 out]
        n119 = Enqueue Element(queue=w256, element=HMI_State."Go to Diagnostics Page", error in (no error)=w257) -> (error out=w254:errorcluster)  [unwired: 1 in, 2 out]
      }
      event "Alarms Page": Mouse Down {
        n120 = event-data() -> ()  [unwired: 1 in, 1 out]
        n121 = Enqueue Element(queue=w260, element=HMI_State."Go to Alarms Page", error in (no error)=w261) -> (error out=w258:errorcluster)  [unwired: 1 in, 2 out]
      }
      event "Status Page": Mouse Down {
        n122 = event-data() -> ()  [unwired: 1 in, 1 out]
        n123 = Enqueue Element(queue=w262, element=HMI_State."Go to Status Page", error in (no error)=w264) -> (error out=w263:errorcluster)  [unwired: 1 in, 2 out]
      }
    }
  }
  n124 = while {
    shift-right: [w269] -> w6
    shift-left: w5 -> [w271]
    tunnel: w1 -> [w268]
    stop <- w266 stop-if-true
    # "Consumer"
    n125 = Dequeue Element(queue=w268, error in (no error)=w271) -> (element=w267:T22, error out=w270:errorcluster)  [unwired: 1 in, 2 out]
    n126 = case shown="\"Timeout\", Default" w267 {
      tunnel: w270 -> [w272 w278 w284 w290 w296]
      tunnel: [w272 w278 w284 w290 w296] -> w269
      frame "Timeout", Default {
      }
      frame "Go to Main Page" {
        n127 = local write "Status Page"(FALSE ("Alarms Page")) -> ()
        n128 = local write "Main Page"(TRUE ("Main Page")) -> ()
        n129 = local write "Diagnostics Page"(FALSE ("Diagnostics Page")) -> ()
        n130 = local write "Alarms Page"(FALSE ("Alarms Page")) -> ()
        n131 = local write "Tab Control"(HMI_Tab."Main" ("Tab Control")) -> ()
      }
      frame "Go to Status Page" {
        n132 = local write "Main Page"(FALSE ("Main Page")) -> ()
        n133 = local write "Diagnostics Page"(FALSE ("Diagnostics Page")) -> ()
        n134 = local write "Alarms Page"(FALSE ("Alarms Page")) -> ()
        n135 = local write "Status Page"(TRUE ("Alarms Page")) -> ()
        n136 = local write "Tab Control"(HMI_Tab."Status" ("Tab Control")) -> ()
      }
      frame "Go to Diagnostics Page" {
        n137 = local write "Status Page"(FALSE ("Alarms Page")) -> ()
        n138 = local write "Main Page"(FALSE ("Main Page")) -> ()
        n139 = local write "Diagnostics Page"(TRUE ("Diagnostics Page")) -> ()
        n140 = local write "Alarms Page"(FALSE ("Alarms Page")) -> ()
        n141 = local write "Tab Control"(HMI_Tab."Diagnostics" ("Tab Control")) -> ()
      }
      frame "Go to Alarms Page" {
        n142 = local write "Status Page"(FALSE ("Alarms Page")) -> ()
        n143 = local write "Main Page"(FALSE ("Main Page")) -> ()
        n144 = local write "Diagnostics Page"(FALSE ("Diagnostics Page")) -> ()
        n145 = local write "Alarms Page"(TRUE ("Alarms Page")) -> ()
        n146 = local write "Tab Control"(HMI_Tab."Alarms" ("Tab Control")) -> ()
      }
    }
    n147 = local read "Exit Program"() -> (w266:bool)
  }
  n148 = while {
    shift-right: [w302] -> w13
    shift-left: w5 -> [w301]
    shift-right: [w309] -> w14
    shift-left: _ -> [w308]
    shift-right: [w310] -> _
    shift-left: LogState."Open File" ("Log State Out") -> [w307]
    shift-right: [w311] -> w12
    shift-left: _ -> [w306]
    tunnel: string[] ["Time", "Event Name", "Event Description"] ("Channel Names In") -> [w305]
    tunnel: w3 -> [w303]
    stop <- w312 stop-if-true
    # "Event Log"
    n149 = Wait (ms)(milliseconds to wait=u32 100) -> ()  [unwired: 1 out]
    n150 = local read "Clear Alarms"() -> (w300:bool)
    n151 = call "DataLogger.vi"("File Ref In"=w308, "Queue In"=w303, "# Samples to Write"=0, "Clear Error"=w300, "Log State In"=w307, "String Path In"=w306, "Error In"=w301, "Channel Names In"=w305, "File Name"="EventLog") -> ("File Ref Out"=w309:refnum<file>, "Log State Out"=w310:T20, "String Path Out"=w311:string, "Error Out"=w302:errorcluster)  [unwired: 3 in]
    n152 = Unbundle By Name(w302) -> ("status"=→"Event Log Error":bool)
    n153 = local read "Exit Program"() -> (w312:bool)
  }
  n154 = while {
    shift-right: [w317] -> w9
    shift-left: w5 -> [w327]
    shift-right: [w324] -> w7
    shift-left: _ -> [w323]
    shift-right: [w325] -> _
    shift-left: LogState."Open File" ("Log State Out") -> [w322]
    shift-right: [w326] -> w8
    shift-left: _ -> [w321]
    tunnel: string[] ["Time", "SSG AC Current", "SSG AC Voltage", "SSG Active Power", "SSG Reactive Power", "SSG Apparent Power", "SSG Frequency", "ES SOC", "ES SOH", "ES Voltage", "ES # Strings", "ES # Cycles", "ES Temperature", "PC Temperature", "Solar Active Power", "Gen W Run Hours", "Gen W Battery Voltage", "Gen W Fuel Rate", "Gen W Total Fuel", "Gen W Power Factor", "Gen W Active Power", "Gen W Reactive Power", "Gen W Apparent Power", "Gen W Frequency", "Gen E Run Hours", "Gen E Battery Voltage", "Gen E Fuel Rate", "Gen E Total Fuel", "Gen E Power Factor", "Gen E Active Power", "Gen E Reactive Power", "Gen E Apparent Power", "Gen E Frequency", "Software Revision", "System Status", "System Faults", "Controller Faults", "ES System Faults", "ES System Alarms", "Converter Faults", "Solar Faults", "ES Rack 1 Faults", "ES Rack 2 Faults", "ES Rack 3 Faults", "ES Rack 4 Faults", "ES Rack 5 Faults", "ES Rack 6 Faults", "ES Rack 7 Faults", "ES Rack 8 Faults", "ES Rack 9 Faults", "ES Rack 10 Faults", "ES Rack 1 Alarms", "ES Rack 2 Alarms", "ES Rack 3 Alarms", "ES Rack 4 Alarms", "ES Rack 5 Alarms", "ES Rack 6 Alarms", "ES Rack 7 Alarms", "ES Rack 8 Alarms", "ES Rack 9 Alarms", "ES Rack 10 Alarms"] ("Channel Names In") -> [w320]
    tunnel: w4 -> [w318]
    stop <- w328 stop-if-true
    # "Data Log"
    n155 = Wait (ms)(milliseconds to wait=u32 100) -> ()  [unwired: 1 out]
    n156 = local read "Clear Alarms"() -> (w315:bool)
    n157 = call "DataLogger.vi"("File Ref In"=w323, "Queue In"=w318, "# Samples to Write"=1, "Clear Error"=w315, "Log State In"=w322, "String Path In"=w321, "Error In"=w327, "Channel Names In"=w320, "File Name"="DataLog") -> ("File Ref Out"=w324:refnum<file>, "Log State Out"=w325:T20, "String Path Out"=w326:string, "Error Out"=w317:errorcluster)  [unwired: 3 in]
    n158 = Unbundle By Name(w317) -> ("status"=→"Data Log Error":bool)
    n159 = local read "Exit Program"() -> (w328:bool)
  }
  n160 = while {
    shift-right: [w334] -> _
    shift-left: w5 -> [w331]
    tunnel: w4 -> [w333]
    stop <- w336 stop-if-true
    # "Queue Data Log"
    n161 = Wait Until Next ms Multiple(millisecond multiple=u32 100 ("milliseconds to wait")) -> ()  [unwired: 1 out]
    n162 = call "Elapsed Time"("Time Target (s)"=5.0, "error in (no error)"=w331) -> ("Time has Elapsed"=w329:bool, "error out"=w330:errorcluster)  [unwired: 10 in, 6 out]
    n163 = case shown="True" w329 {
      tunnel: [w337 w343] -> w334
      tunnel: w330 -> [w337 w341]
      tunnel: w333 -> [_ w339]
      frame False {
      }
      frame True {
        n164 = local read "InterfaceData"() -> (w338:T14)
        n165 = call "Data Bundle.vi"("Error In"=w341, "InterfaceData"=w338) -> ("Error Out"=w342:errorcluster, "Data Out"=w340:string[])  [unwired: 8 in]
        n166 = Enqueue Element(queue=w339, element=w340, error in (no error)=w342) -> (error out=w343:errorcluster)  [unwired: 1 in, 2 out]
      }
    }
    n167 = local read "Exit Program"() -> (w336:bool)
  }
  n168 = while {
    shift-right: [w363] -> _
    shift-left: w5 -> [w358]
    shift-right: [w364] -> _
    shift-left: T21 {"Message Array"=[], "Fault Array"=[FALSE, FALSE, FALSE, FALSE, FALSE, FALSE, FALSE, FALSE, FALSE, FALSE, FALSE, FALSE, FALSE, FALSE, FALSE, FALSE], "Alarm Array"=[FALSE, FALSE, FALSE, FALSE, FALSE, FALSE, FALSE, FALSE, FALSE, FALSE, FALSE, FALSE, FALSE, FALSE, FALSE, FALSE]} ("Alarms Cluster") -> [w356]
    stop <- w368 stop-if-true
    w357 = 1.0 ("Time Target (s)")
    # "Manage Alarms"
    n169 = Wait (ms)(milliseconds to wait=u32 100) -> ()  [unwired: 1 out]
    n170 = local read "Connection Error"() -> (w353:bool)
    n171 = local read "Event Log Error"() -> (w350:bool)
    n172 = local read "Data Log Error"() -> (w349:bool)
    n173 = local read "InterfaceData"() -> (w344:T14)
    n174 = Compound Arithmetic op=OR(w350, w349) -> (w348:bool)
    n175 = call "Alarms Read.vi"("Error In"=w358, "InterfaceData"=w344, "Alarms Data In"=w356) -> ("Error Out"=w367:errorcluster, "Alarms Data Out"=w366:T21)  [unwired: 7 in]
    n176 = call "Alarms Clear.vi"("Clear Alarms In"="Clear Alarms", "Error In"=w367, "Alarms Data In"=w366) -> ("Error Out"=w365:errorcluster, "Alarms Data Out"=w364:T21)  [unwired: 7 in]
    n177 = feedback-in #1("Clear Alarms") -> ()
    n178 = feedback #1(FALSE ("Clear Alarms")) -> (w347:bool)
    n179 = call "Wait Timer.vi"("Boolean In"=w347, "Timer"=u32 2) -> ("Boolean Out"=w346:bool)  [unwired: 3 in]
    n180 = call "Alarms Display.vi"("Alarm Input"=w348, "Fault Input"=w353, "Error In"=w365, "Alarms Data In"=w364) -> ("Error Out"=w363:errorcluster, "Alarm?"=w362:bool, "Fault?"=w352:bool, "Alarm List"=→"Alarms List":T16)  [unwired: 4 in]
    n181 = case shown="True" w346 {
      frame False {
      }
      frame True {
        n182 = local write "Clear Alarms"(FALSE ("Clear Alarms")) -> ()
      }
    }
    n183 = Compound Arithmetic op=AND(invert w352, w362) -> (w361:bool)
    n184 = call "Pulse Output.vi"("Boolean In"=w352, "Time Target (s)"=w357) -> ("Boolean Out"=→"Fault Banner":bool)  [unwired: 3 in]
    n185 = call "Pulse Output.vi"("Boolean In"=w361, "Time Target (s)"=w357) -> ("Boolean Out"=→"Alarm Banner":bool)  [unwired: 3 in]
    n186 = local read "Exit Program"() -> (w368:bool)
  }
  n187 = Release Queue(queue=w1, error in (no error)=w6) -> ()  [unwired: 1 in, 3 out]
  n188 = call "DataLogger.vi"("File Ref In"=w7, "Queue In"=w4, "Log State In"=LogState."Close File", "String Path In"=w8, "Error In"=w9) -> ("Error Out"=w10:errorcluster)  [unwired: 7 in, 3 out]
  n189 = Release Queue(queue=w4, error in (no error)=w10) -> ()  [unwired: 1 in, 3 out]
  n190 = call "QueueEvent.vi"("Error In"=w13, "Event Description"="HMI Shutdown", "Event Name"="State", "Queue In"=w3) -> ("Error Out"=w19:errorcluster, "Queue Out"=w16:refnum<queue>)  [unwired: 6 in]
  n191 = call "DataLogger.vi"("File Ref In"=w14, "Queue In"=w16, "Log State In"=LogState."Close File", "String Path In"=w12, "Error In"=w19) -> ("Error Out"=w20:errorcluster)  [unwired: 7 in, 3 out]
  n192 = Release Queue(queue=w16, error in (no error)=w20) -> ()  [unwired: 1 in, 3 out]
